vi "已用时间定时器.vi"(8 "error in":errorcluster, 10 "reset mode":bool, 11 "reset":bool) -> (0 "error out":errorcluster, 3 "elapsed time (ms)":i32)   [LabVIEW 2012, in "毫秒定时器.lvlib"]
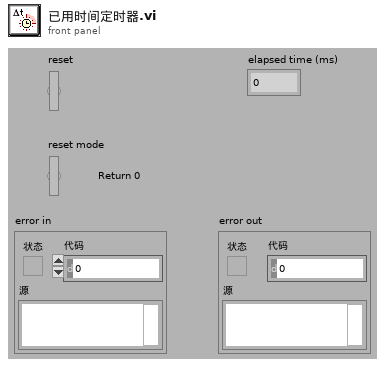
[diagram p1: front panel]
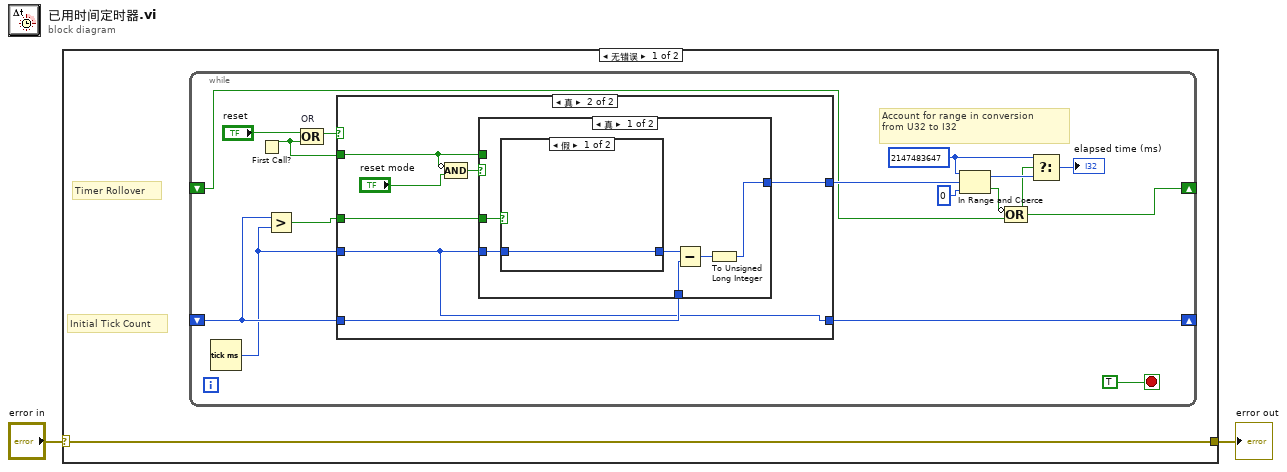
[diagram p0: block diagram]
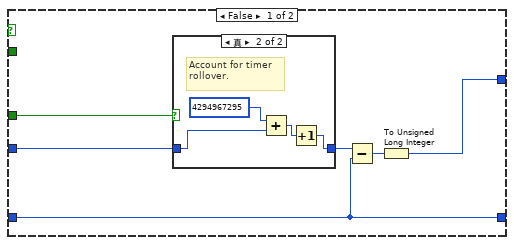
[diagram p2: hidden frame]
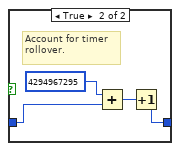
[diagram p4: hidden frame]
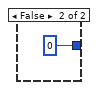
[diagram p5: hidden frame]
diagram:
  n1 = case shown="无错误" "error in" {
    selector: "error in" -> [w3 w50]
    tunnel: [w3 w50] -> w1
    frame No Error {
      # "Initial Tick Count"
      # "Timer Rollover"
      n2 = while {
        shift-right: [w5] -> _
        shift-left: _ -> [w6]
        shift-right: [w9] -> _
        shift-left: _ -> [w7]
        stop <- TRUE stop-if-true
        w10 = u32 2147483647 ("upper limit")
        # "Account for range in conversion\nfrom U32 to I32"
        n3 = Tick Count (ms)() -> (millisecond timer value=w4:u32)
        n4 = First Call?() -> (First Call?: T/F=w16:bool)
        n5 = Greater?(x=w7, y=w4) -> (0:w8:bool)
        n6 = Compound Arithmetic op=OR "OR"("reset", w16) -> (w18:bool)
        n7 = case shown="真" w18 {
          tunnel: [w21 w37] -> w14
          tunnel: w16 -> [_ w36]
          tunnel: w8 -> [w24 w33]
          tunnel: w4 -> [w23 w31]
          tunnel: [w20 w31] -> w9
          tunnel: w7 -> [w20 w32]
          frame False {
            n8 = case shown="真" w24 {
              tunnel: w23 -> [w26 w29]
              tunnel: [w26 w28] -> w22
              frame False {
              }
              frame True {
                # "Account for timer rollover."
                n9 = Add(x=u64 4294967295, y=w29) -> (x+y=w27:u64)
                n10 = Increment(x=w27) -> (x+1=w28:u64)
              }
            }
            n11 = Subtract(x=w22, y=w20) -> (x-y=w25:u64)
            n12 = To Unsigned Long Integer(number=w25) -> (unsigned 32bit integer=w21:u32)
          }
          frame True {
            n13 = Compound Arithmetic op=AND(invert w36, "reset mode") -> (w34:bool)
            n14 = case shown="真" w34 {
              tunnel: [w39 u32 0] -> w37
              tunnel: w36 -> [_ _]
              tunnel: w33 -> [w38 _]
              tunnel: w31 -> [w41 _]
              tunnel: w32 -> [w40 _]
              frame True {
                n15 = case shown="假" w38 {
                  tunnel: w41 -> [w44 w47]
                  tunnel: [w44 w45] -> w42
                  frame False {
                  }
                  frame True {
                    # "Account for timer rollover."
                    n16 = Add(x=u64 4294967295, y=w47) -> (x+y=w46:u64)
                    n17 = Increment(x=w46) -> (x+1=w45:u64)
                  }
                }
                n18 = Subtract(x=w42, y=w40) -> (x-y=w43:u64)
                n19 = To Unsigned Long Integer(number=w43) -> (unsigned 32bit integer=w39:u32)
              }
              frame False {
              }
            }
          }
        }
        n20 = In Range and Coerce(upper limit=w10, x=w14, lower limit=u32 0) -> (coerced(x)=w11:u32, In Range?=w13:bool)
        n21 = Compound Arithmetic op=OR(invert w13, w6) -> (w5:bool)
        n22 = Select(t=w10, s=w5, f=w11) -> (s? t:f=→"elapsed time (ms)":u32)
      }
    }
    frame Error {
    }
  }
  "error out" <- w1
